vi "I16_Data To ASCII String.vi"(8 "error in":errorcluster, 11 "Data":i16) -> (0 "error out":errorcluster, 3 "Value":string)   [LabVIEW 2016, in "CVT.lvlib" / "Current Value Table.lvlib"]
doc: "This VI takes data and converts it into an ASCII string. This VI must perform the opposite operation to the ASCIIStringToData function."
uses:
  <vilib>/NI/Current Value Table/Current Value Table.lvlib
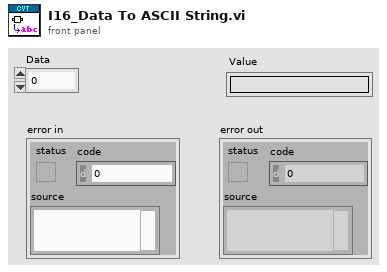
[diagram p1: front panel]
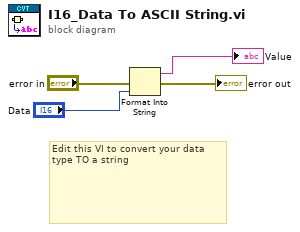
[diagram p0: block diagram]
diagram:
  # "Edit this VI to convert your data type TO a string"
  n1 = Format Into String(error in="error in", "Data") -> (resulting string=→"Value":string, error out=→"error out":errorcluster)  [unwired: 2 in]
